vi "Verify.vi"(7 "Actor":refnum<class "Actor.lvclass">) -> (3 "Stats":T1)   [LabVIEW 2020, in "_Template.lvlib" / "{{Actor}}.lvlib" / "Actor.lvclass"]
uses:
  Actor.lvclass
  Actor.lvclass/Actor.ctl
  jettl/jettl/jettl.lvlib
  jettl/jettl/MsgNames.ctl
  jettl/jettl/Stats.ctl
panel:
  # "This front panel should not be manipulated."
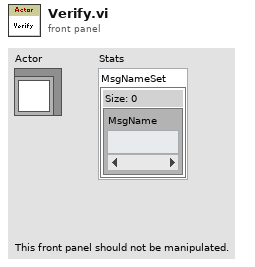
[diagram p1: front panel]
types:
  T1 = typedef "jettl.lvlib/Stats.ctl" = cluster{"MsgNameSet":T2}
  T2 = typedef "jettl.lvlib/MsgNames.ctl" = set{string}
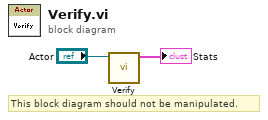
[diagram p0: block diagram]
diagram:
  # "This block diagram should not be manipulated."
  n1 = call "Verify.vi"("Actor.lvclass"="Actor") -> ("Stats"=→"Stats":T1)  [unwired: 10 in]
